vi "Configure Error Mode.vi"(8 "error in (no error)":errorcluster, 9 "Error Unit (0: Threshold 1000)":i32(ring) items=["Threshold 1000", "Threshold 100", "Threshold 10", "Parts-per-million", "Percent"], 10 "Edit Field Type (0: Primary)":i32(ring) items=["Primary", "Secondary", "Frequency"], 11 "VISA resource name":refnum<visa-resource-name>) -> (0 "error out":errorcluster, 3 "VISA resource name out":refnum<visa-resource-name>)   [LabVIEW 2012, in "Fluke 5080.lvlib"]
doc: "Configures the error unit."
uses:
  <instrlib>/Fluke 5080/Fluke 5080.lvlib
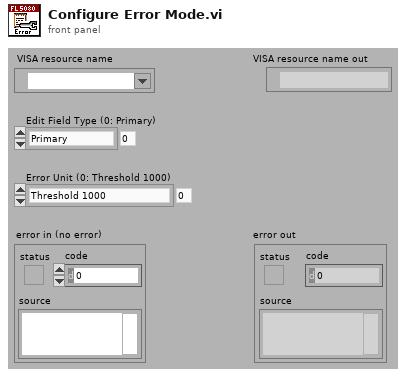
[diagram p1: front panel]
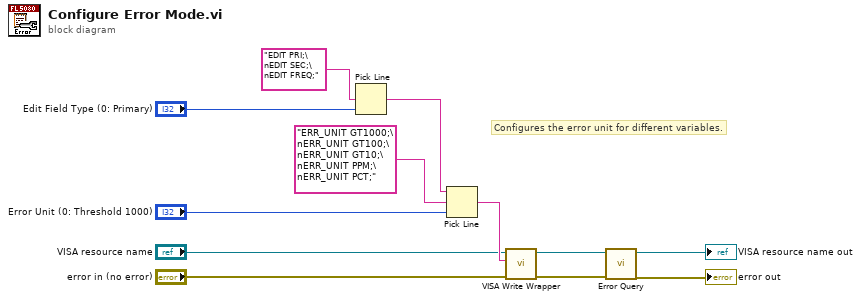
[diagram p0: block diagram]
diagram:
  # "Configures the error unit for different variables."
  n1 = Pick Line(multi-line string="EDIT PRI;\nEDIT SEC;\nEDIT FREQ;", line index="Edit Field Type (0: Primary)") -> (output string=w8:string)  [unwired: 1 out]
  n2 = Pick Line(string ("")=w8, multi-line string="ERR_UNIT GT1000;\nERR_UNIT GT100;\nERR_UNIT GT10;\nERR_UNIT PPM;\nERR_UNIT PCT;", line index="Error Unit (0: Threshold 1000)") -> (output string=w7:string)
  n3 = call <instrlib>:"VISA Write Wrapper.vi"("error in (no error)"="error in (no error)", "Write Buffer"=w7, "VISA resource name"="VISA resource name") -> ("error out"=w3:errorcluster, "VISA resource name out"=w4:refnum<visa-resource-name>)  [unwired: 7 out]
  n4 = call <instrlib>:"Error Query.vi"("error in (no error)"=w3, "VISA resource name"=w4) -> ("error out"=→"error out":errorcluster, "VISA resource name out"=→"VISA resource name out":refnum<visa-resource-name>)  [unwired: 8 out]
